vi "Read Color.vi"(8 "error in (no error)":errorcluster, 11 "Shape in":refnum<class "Shape.lvclass">) -> (0 "error out":errorcluster, 2 "Color":u32(colorbox), 3 "Shape out":refnum<class "Shape.lvclass">)   [LabVIEW 2015, in "LV Image Editor Framework.lvlib" / "Shape.lvclass"]
uses:
  Shape.lvclass
  Shape.lvclass/Shape.ctl
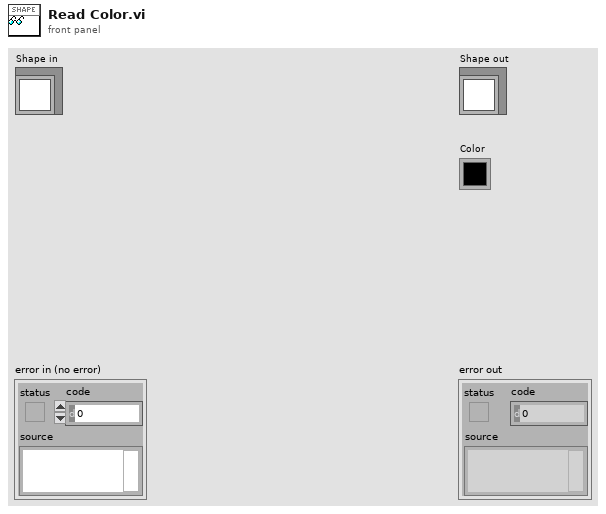
[diagram p1: front panel]
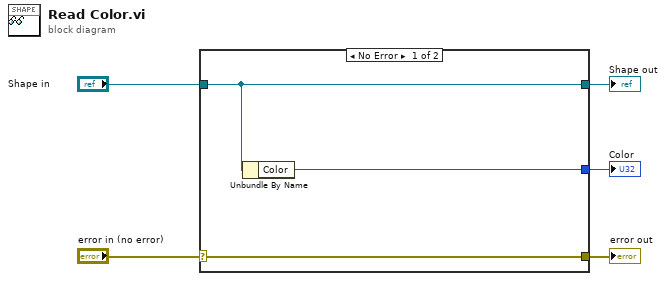
[diagram p0: block diagram]
diagram:
  n1 = case shown="No Error" "error in (no error)" {
    selector: "error in (no error)" -> [w8 w9]
    tunnel: [w8 w9] -> w4
    tunnel: [w7 w10] -> w2
    tunnel: "Shape in" -> [w7 w10]
    tunnel: [w6 _] -> w1
    frame No Error {
      n2 = Unbundle By Name(w7) -> ("Color"=w6:u32)
    }
    frame Error {
    }
  }
  "error out" <- w4
  "Shape out" <- w2
  "Color" <- w1
